vi "Set Blueprint.vi"(8 "error in (no error)":errorcluster, 10 "Blueprint":refnum<class "Blueprint.lvclass">, 11 "BP Summary in":refnum<class "BP Summary.lvclass">) -> (0 "error out":errorcluster, 3 "BP Summary out":refnum<class "BP Summary.lvclass">)   [LabVIEW 2020, in "BP Summary.lvclass"]
uses:
  BP Summary.lvclass
  Blueprint/Blueprint.lvclass
  BP Summary.lvclass/BP Summary.ctl
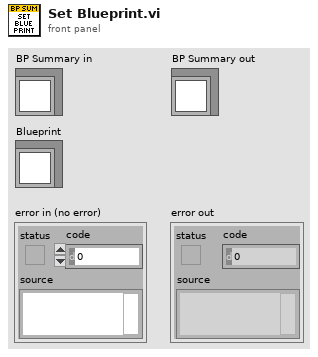
[diagram p1: front panel]
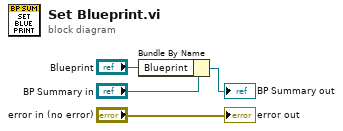
[diagram p0: block diagram]
diagram:
  n1 = Bundle By Name(cluster="BP Summary in", "Blueprint"="Blueprint") -> (→"BP Summary out":refnum<class "BP Summary.lvclass">)
  "error out" <- "error in (no error)"
